vi "PictureCounter.vi"(5 "Reset? (f)":bool, 7 "count? (T)":bool=TRUE) -> (2 "y":u16, 3 "x":u16)   [LabVIEW 2019, in "Shared.lvlib"]
uses:
  Shared.lvlib
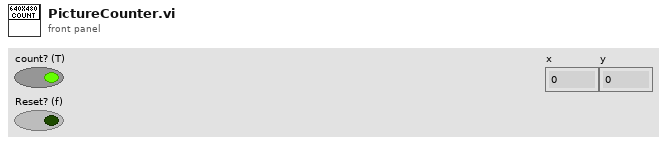
[diagram p1: front panel]
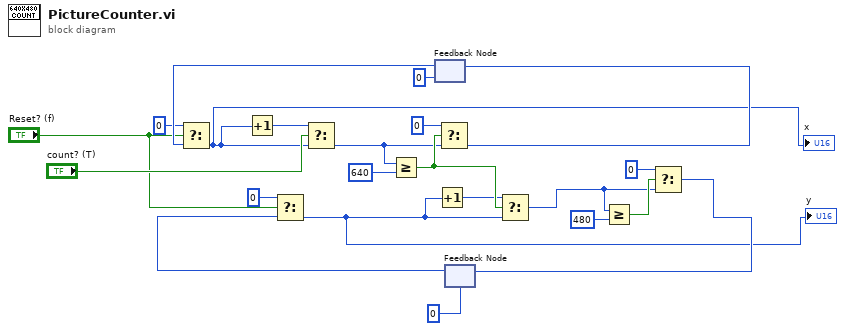
[diagram p0: block diagram]
diagram:
  n1 = feedback #1(u16 0 ("t")) -> (w7:u16)
  n2 = Select(t=u16 0, s="Reset? (f)", f=w7) -> (s? t:f=w5:u16)
  "x" <- w5
  n3 = Increment(x=w5) -> (x+1=w10:u16)
  n4 = Select(t=w10, s="count? (T)", f=w5) -> (s? t:f=w11:u16)
  n5 = Greater Or Equal?(x=w11, y=u16 640) -> (x >= y?=w19:bool)
  n6 = Select(t=u16 0, s=w19, f=w11) -> (s? t:f=w22:u16)
  n7 = feedback-in #1(w22) -> ()
  n8 = feedback #2(u16 0 ("t")) -> (w6:u16)
  n9 = Select(t=u16 0, s="Reset? (f)", f=w6) -> (s? t:f=w1:u16)
  "y" <- w1
  n10 = Increment(x=w1) -> (x+1=w18:u16)
  n11 = Select(t=w18, s=w19, f=w1) -> (s? t:f=w12:u16)
  n12 = Greater Or Equal?(x=w12, y=u16 480) -> (x >= y?=w15:bool)
  n13 = Select(t=u16 0, s=w15, f=w12) -> (s? t:f=w21:u16)
  n14 = feedback-in #2(w21) -> ()
